vi "Launch.vi"(9 "Alias":string, 10 "Actor":refnum<class "Actor.lvclass">) -> (0 "error out":errorcluster)   [LabVIEW 2021]
uses:
  <vilib>/jettl/jettl/jettl/Actor/Actor.lvclass
  <vilib>/jettl/jettl/jettl/Self Actor/Create Top Level.vi
  <vilib>/jettl/jettl/jettl/Self Actor/Self Actor.lvclass
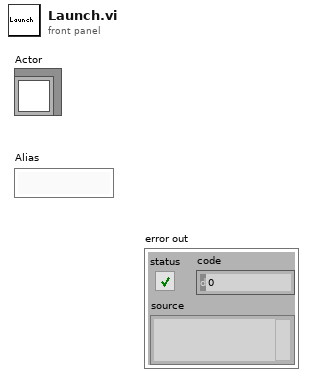
[diagram p1: front panel]
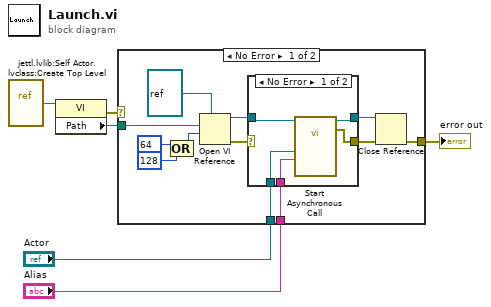
[diagram p0: block diagram]
diagram:
  n1 = vi-ref "jettl.lvlib:Self Actor.lvclass:Create Top Level.vi"() -> (w5:refnum<vi>)
  n2 = property class="VI"(reference=w5) -> (error out=w6:errorcluster, "Path"=w4:path)  [unwired: 1 in, 1 out]
  n3 = case shown="No Error" w6 {
    selector: w6 -> [_ w26]
    tunnel: [w16 w26] -> w2
    tunnel: w4 -> [w12 _]
    tunnel: "Actor" -> [w8 _]
    tunnel: "Alias" -> [w7 _]
    frame No Error {
      n4 = Compound Arithmetic op=OR(64 ("options: Multiple Clones,\n  Fire & Forget"), 128 ("options: Multiple Clones,\n  Fire & Forget")) -> (w14:i32)
      n5 = Open VI Reference(type specifier VI Refnum (for type only)=refnum<vi> refnum, vi path=w12, options=w14) -> (vi reference=w10:refnum<vi>, error out=w11:errorcluster)  [unwired: 3 in]
      n6 = case shown="No Error" w11 {
        selector: w11 -> [_ w25]
        tunnel: [w22 w24] -> w18
        tunnel: [w21 w25] -> w17
        tunnel: w10 -> [w23 w24]
        tunnel: w8 -> [w20 _]
        tunnel: w7 -> [w19 _]
        frame No Error {
          n7 = call-by-ref "Start Asynchronous Call"(reference=w23, "Alias"=w19, "Actor"=w20) -> (reference out=w22:refnum<vi>, error out=w21:errorcluster)  [unwired: 11 in]
        }
        frame Error {
        }
      }
      n8 = Close Reference(reference=w18, error in (no error)=w17) -> (error out=w16:errorcluster)
    }
    frame Error {
    }
  }
  "error out" <- w2
